vi "gfitsio-read-image-subset.vi"   [LabVIEW 2022 SP3, in "gfitsio.lvlib"]
uses:
  <userlib>/gfitsio/gfitsio.lvlib
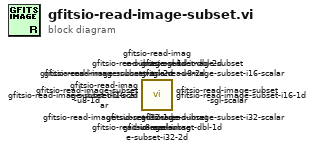
[diagram p0: block diagram]
diagram:
  n1 = call <userlib>:"gfitsio-read-image-subset-u8-scalar.vi"() -> ()  [unwired: 9 in, 3 out]
  n2 = call <userlib>:"gfitsio-read-image-subset-u8-2d.vi"() -> ()  [unwired: 9 in, 3 out]
  n3 = call <userlib>:"gfitsio-read-image-subset-u8-1d.vi"() -> ()  [unwired: 9 in, 3 out]
  n4 = call <userlib>:"gfitsio-read-image-subset-sgl-scalar.vi"() -> ()  [unwired: 9 in, 3 out]
  n5 = call <userlib>:"gfitsio-read-image-subset-sgl-2d.vi"() -> ()  [unwired: 9 in, 3 out]
  n6 = call <userlib>:"gfitsio-read-image-subset-sgl-1d.vi"() -> ()  [unwired: 9 in, 3 out]
  n7 = call <userlib>:"gfitsio-read-image-subset-i32-scalar.vi"() -> ()  [unwired: 9 in, 3 out]
  n8 = call <userlib>:"gfitsio-read-image-subset-i32-2d.vi"() -> ()  [unwired: 9 in, 3 out]
  n9 = call <userlib>:"gfitsio-read-image-subset-i32-1d.vi"() -> ()  [unwired: 9 in, 3 out]
  n10 = call <userlib>:"gfitsio-read-image-subset-i16-2d.vi"() -> ()  [unwired: 9 in, 3 out]
  n11 = call <userlib>:"gfitsio-read-image-subset-i16-1d.vi"() -> ()  [unwired: 9 in, 3 out]
  n12 = call <userlib>:"gfitsio-read-image-subset-i16-scalar.vi"() -> ()  [unwired: 9 in, 3 out]
  n13 = call <userlib>:"gfitsio-read-image-subset-dbl-2d.vi"() -> ()  [unwired: 9 in, 3 out]
  n14 = call <userlib>:"gfitsio-read-image-subset-dbl-1d.vi"() -> ()  [unwired: 9 in, 3 out]
  n15 = call <userlib>:"gfitsio-read-image-subset-variant.vi"() -> ()  [unwired: 9 in, 3 out]
  n16 = call <userlib>:"gfitsio-read-image-subset-dbl-scalar.vi"() -> ()  [unwired: 9 in, 3 out]
